vi "Convert Percent to Flow Rate.vi"(10 "Flow Rate Constant":dbl format="%#_13g", 11 "New Parameters (percents)":T1) -> (2 "New Parameters (values) out":T1, 3 "New Parameters (percents) out":T1)   [LabVIEW 2020, in "Deep Reaction Optimizer Control Panel.lvlib" / "Instrument Manager.lvlib"]
uses:
  Instrument Manager.lvlib
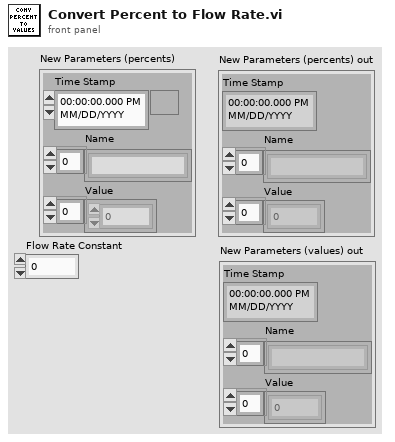
[diagram p1: front panel]
types:
  T1 = cluster{"Time Stamp":timestamp, "Name":string[], "Value":dbl[]}
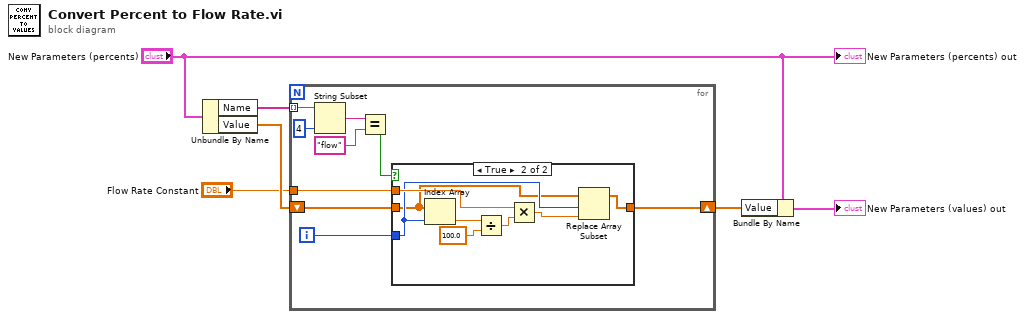
[diagram p0: block diagram]
diagram:
  n1 = Unbundle By Name("New Parameters (percents)") -> ("Name"=w6:string[], "Value"=w5:dbl[])
  n2 = for {
    tunnel: w6 -> [w15] mode=indexing
    shift-right: [w8] -> w2
    shift-left: w5 -> [w9]
    tunnel: "Flow Rate Constant" -> [w11]
    i -> [w10]
    n3 = String Subset(string=w15, length (rest)=4 ("length (rest)")) -> (substring=w13:string)  [unwired: 1 in]
    n4 = Equal?(x=w13, y="flow") -> (x = y?=w7:bool)
    n5 = case shown="True" w7 {
      tunnel: w11 -> [_ w22]
      tunnel: w10 -> [_ w20]
      tunnel: w9 -> [w16 w19]
      tunnel: [w16 w18] -> w8
      frame False {
      }
      frame True {
        n6 = Index Array(array=w19, index=w20) -> (element=w24:dbl)
        n7 = Divide(x=w24, y=100.0) -> (x/y=w21:dbl)
        n8 = Multiply(x=w22, y=w21) -> (x*y=w17:dbl)
        n9 = Replace Array Subset(array=w19, new element=w17, index=w20) -> (w18:dbl[])
      }
    }
  }
  n10 = Bundle By Name(cluster="New Parameters (percents)", "Value"=w2) -> (→"New Parameters (values) out":T1)
  "New Parameters (percents) out" <- "New Parameters (percents)"
